vi "Add Node.vi"(6 "T: Ignore Repeat Root":bool, 7 "Parent Path":string, 8 "Attributes":map{string, string}(c390), 9 "Data":string, 10 "New Node Name":string, 11 "Tree Map In":T1) -> (0 "Path Invalid":bool, 3 "Tree Map Out":T1, 5 "New Node Path":string)   [LabVIEW 2021, in "Tree Map.lvlib"]
doc: "Add a node to the Tree Map. Data asociated with this node can be optionally specified.\n\n<b>NOTE</b> Be careful not to use XML special characters for the data or name of the node if you intend to flatten and unflatten from XML. This can cause error in XML functions.\n\n<b>Author:</b> Piotr Kruczkowski <PrimaryKey>\n<b>License:</b> NewBSD\n\nCopyright (c) 2019, National Instruments\nAll rights reserved.\n\nRedistribution and use in source and binary forms, with or without\nmodification, are permitted provided that the following conditions are met:\n1. Redistributions of source code must retain the above copyright\n notice, this list of conditions and the following disclaimer.\n2. Redistributions in binary form must reproduce the above copyright\n notice, this list of conditions and the following disclaimer in the\n documentation and/or other materials provided with the distribution.\n3. Neither the name of National Instruments nor the\n names of its contributors may be used to endorse or promote products\n derived from this software without specific prior written permission.\n\nTHIS SOFTWARE IS PROVIDED BY National Instruments ''AS IS'' AND ANY\nEXPRESS OR IMPLIED WARRANTIES, INCLUDING, BUT NOT LIMITED TO, THE IMPLIED\nWARRANTIES OF MERCHANTABILITY AND FITNESS FOR A PARTICULAR PURPOSE ARE\nDISCLAIMED. IN NO EVENT SHALL National Instruments BE LIABLE FOR ANY\nDIRECT, INDIRECT, INCIDENTAL, SPECIAL, EXEMPLARY, OR CONSEQUENTIAL DAMAGES\n(INCLUDING, BUT NOT LIMITED TO, PROCUREMENT OF SUBSTITUTE GOODS OR SERVICES;\nLOSS OF USE, DATA, OR PROFITS; OR BUSINESS INTERRUPTION) HOWEVER CAUSED AND\nON ANY THEORY OF LIABILITY, WHETHER IN CONTRACT, STRICT LIABILITY, OR TORT\n(INCLUDING NEGLIGENCE OR OTHERWISE) ARISING IN ANY WAY OUT OF THE USE OF THIS\nSOFTWARE, EVEN IF ADVISED OF THE POSSIBILITY OF SUCH DAMAGE."
uses:
  <vilib>/National Instruments/Tree Map/Tree Map.lvlib
  <vilib>/National Instruments/Tree Map/Tree Map Data.ctl
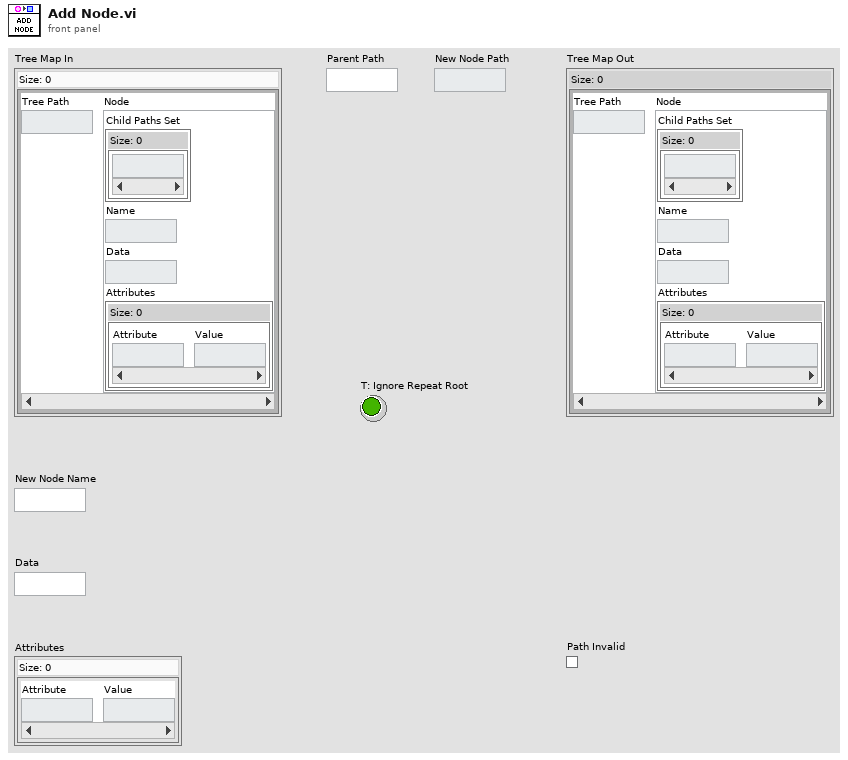
[diagram p1: front panel]
types:
  T1 = typedef "Tree Map.lvlib/Tree Map Data.ctl" = map{string, cluster{"Child Paths Set":set{string}, "Name":string, "Data":string, "Attributes":map{string, string}}}
  T2 = cluster{"Child Paths Set":set{string}, "Name":string, "Data":string, "Attributes":map{string, string}}
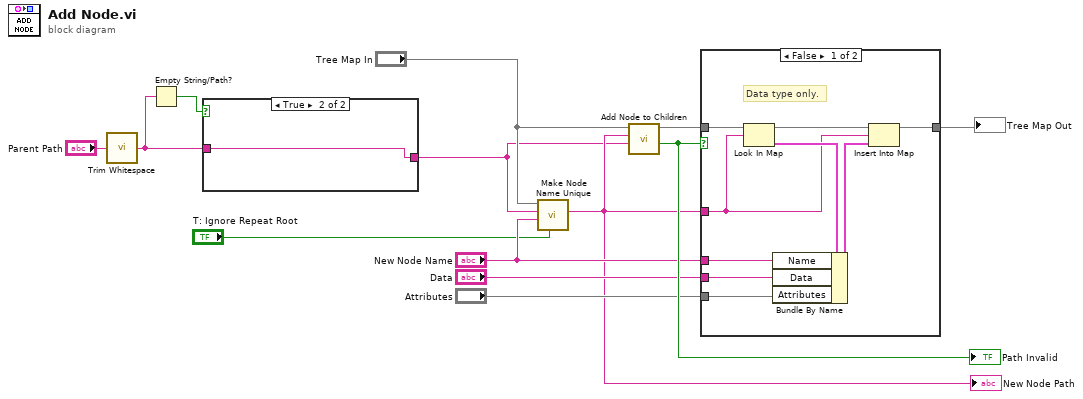
[diagram p0: block diagram]
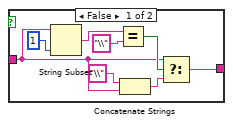
[diagram p2: hidden frame]
diagram:
  n1 = call <vilib>:"Trim Whitespace.vi"("string"="Parent Path") -> ("trimmed string"=w3:string)  [unwired: 1 in]
  n2 = Empty String/Path?(string/path=w3) -> (empty?=w2:bool)
  n3 = case shown="True" w2 {
    tunnel: [w15 w22] -> w4
    tunnel: w3 -> [w14 w22]
    frame False {
      n4 = String Subset(string=w14, length (rest)=1 ("length (rest)")) -> (substring=w19:string)  [unwired: 1 in]
      n5 = Equal?(x=w19, y="\\") -> (x = y?=w17:bool)
      n6 = Concatenate Strings("\\" ("string"), w14) -> (w16:string)
      n7 = Select(t=w14, s=w17, f=w16) -> (s? t:f=w15:string)
    }
    frame True {
    }
  }
  n8 = call <vilib>:"Make Node Name Unique.vi"("T: Ignore Repeat Root"="T: Ignore Repeat Root", "New Node Name"="New Node Name", "Parent Path"=w4, "Tree Map In"="Tree Map In") -> ("Node Path"=w6:string)  [unwired: 6 in, 1 out]
  "New Node Path" <- w6
  n9 = call <vilib>:"Add Node to Children.vi"("Parent Path"=w4, "Node Path"=w6, "Tree Map In"="Tree Map In") -> ("Path Invalid"=w13:bool, "Tree Map Out"=w9:T1)  [unwired: 7 in]
  "Path Invalid" <- w13
  n10 = case shown="False" w13 {
    tunnel: w9 -> [w29 w31]
    tunnel: w6 -> [w26 _]
    tunnel: [w30 w31] -> w11
    tunnel: "Data" -> [w25 _]
    tunnel: "Attributes" -> [w24 _]
    tunnel: "New Node Name" -> [w23 _]
    frame False {
      # "Data type only."
      n11 = Look In Map(map=w29, key=w26) -> (value=w28:T2)  [unwired: 1 in, 1 out]
      n12 = Bundle By Name(cluster=w28, "Name"=w23, "Data"=w25, "Attributes"=w24) -> (w27:T2)
      n13 = Insert Into Map(map in=w29, key=w26, value=w27) -> (map out=w30:T1)  [unwired: 2 out]
    }
    frame True {
    }
  }
  "Tree Map Out" <- w11
